vi "仪器版本写入.vi"(8 "error in (no error)":errorcluster caption="错误输入（无错误）", 10 "仪器版本":T1, 11 "SingleStepTestV3 输入":refnum<class "SingleStepTestV3.lvclass">) -> (0 "error out":errorcluster caption="错误输出", 3 "SingleStepTestV3 输出":refnum<class "SingleStepTestV3.lvclass">)   [LabVIEW 2022 SP3, in "SingleStepTestV3.lvlib" / "SingleStepTestV3.lvclass"]
uses:
  SingleStepTestV3.lvclass
  SingleStepTestV3.lvclass/SingleStepTestV3.ctl
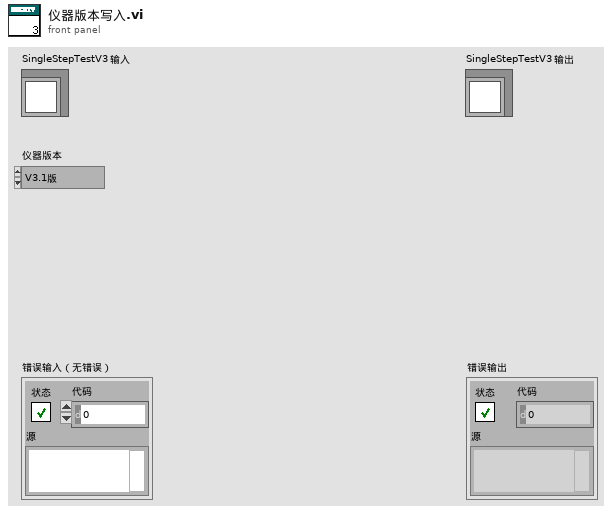
[diagram p1: front panel]
types:
  T1 = typedef "SingleStepTestV3.lvlib/SingleStepTestV3.lvclass/仪器版本.ctl" = enum16{"V3.1版", "V4版", "V3版", "V4.2版"}
  T2 = typedef "SingleStepTestV3.lvlib/SingleStepTestV3.lvclass/State Data.ctl" = cluster{"data":u16[], "仪器版本":T1}
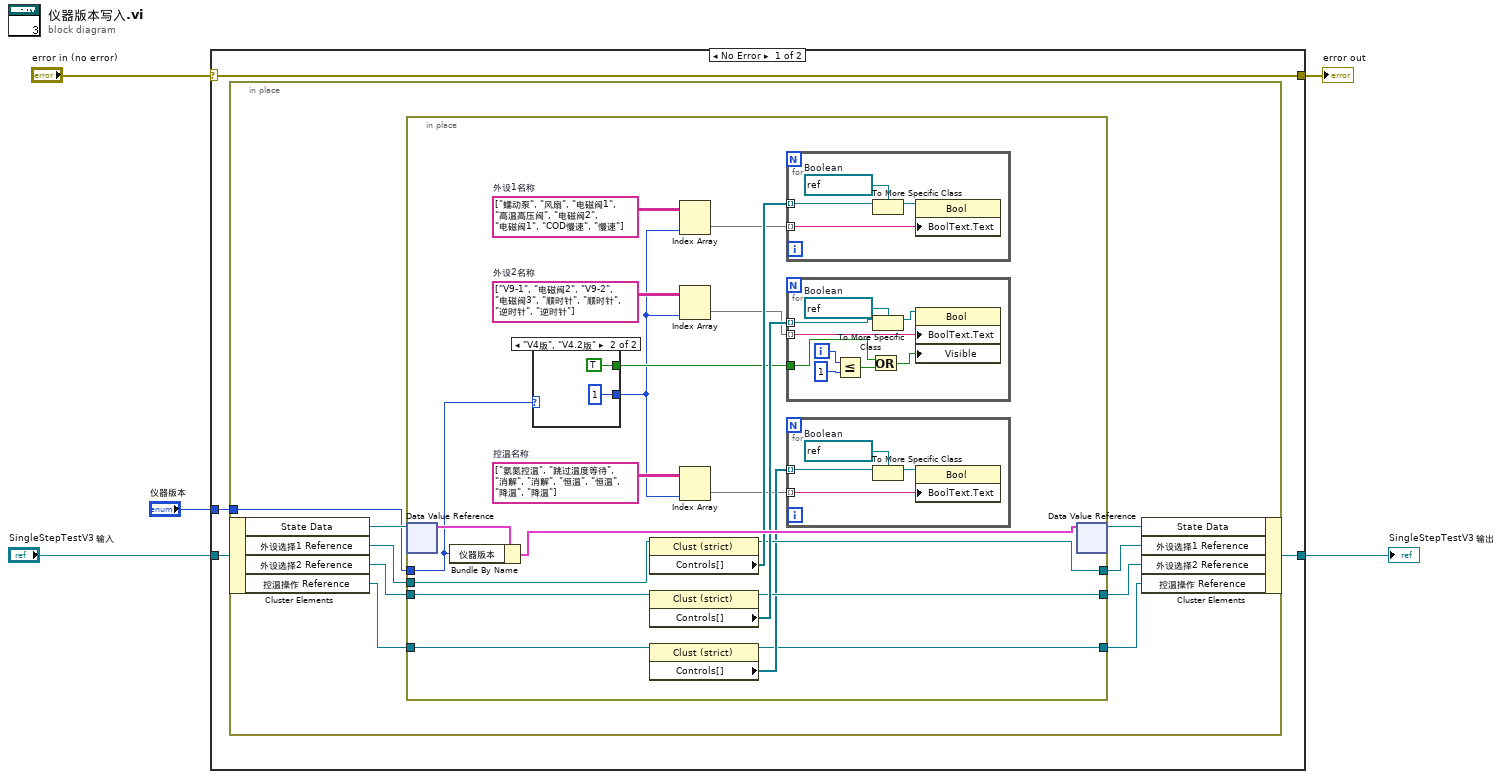
[diagram p0: block diagram]
diagram:
  n1 = case shown="No Error" "error in (no error)" {
    selector: "error in (no error)" -> [w9 w59]
    tunnel: [w9 w59] -> w4
    tunnel: [w7 w58] -> w2
    tunnel: "SingleStepTestV3 输入" -> [w8 w58]
    tunnel: "仪器版本" -> [w6 _]
    frame No Error {
      n2 = in-place {
        in-place-border: w6 -> [w16]
        n3 = in-place-cluster #1(w8) -> ("State Data"=w18:refnum<data-value>, "外设选择1 Reference"=w15:refnum<vi>, "外设选择2 Reference"=w14:refnum<vi>, "控温操作 Reference"=w11:refnum<vi>)
        n4 = in-place {
          in-place-border: w16 -> [w20]
          in-place-border: w15 -> [w36]
          in-place-border: w14 -> [w35]
          in-place-border: [w28] -> w13
          in-place-border: [w27] -> w12
          in-place-border: w11 -> [w26]
          in-place-border: [w22] -> w10
          w24 = string[][] [["氨氮控温", "跳过温度等待"], ["消解", "消解"], ["恒温", "恒温"], ["降温", "降温"]]  # 控温名称
          w30 = string[][] [["V9-1", "电磁阀2"], ["V9-2", "电磁阀3"], ["顺时针", "顺时针"], ["逆时针", "逆时针"]]  # 外设2名称
          w33 = string[][] [["蠕动泵", "风扇"], ["电磁阀1", "高温高压阀"], ["电磁阀2", "电磁阀1"], ["COD慢速", "慢速"]]  # 外设1名称
          n5 = in-place-dvr #2(w18) -> (w38:T2)  [unwired: 1 out]
          n6 = Bundle By Name(cluster=w38, "仪器版本"=w20) -> (w37:T2)
          n7 = case shown="\"V4版\", \"V4.2版\"" w20 {
            tunnel: [_ TRUE] -> w21
            tunnel: [_ 1] -> w19
            frame "V3.1版", Default {
            }
            frame "V4版", "V4.2版" {
            }
          }
          n8 = property class="Clust (strict)"(reference=w36) -> (reference out=w28:refnum<vi>, "Controls[]"=w34:refnum<vi>[])  [unwired: 1 in, 1 out]
          n9 = property class="Clust (strict)"(reference=w35) -> (reference out=w27:refnum<vi>, "Controls[]"=w31:refnum<vi>[])  [unwired: 1 in, 1 out]
          n10 = property class="Clust (strict)"(reference=w26) -> (reference out=w22:refnum<vi>, "Controls[]"=w25:refnum<vi>[])  [unwired: 1 in, 1 out]
          n11 = Index Array(array=w33, index (col)=w19) -> (element=w32:string[])  [unwired: 1 in]
          n12 = Index Array(array=w30, index (col)=w19) -> (element=w29:string[])  [unwired: 1 in]
          n13 = Index Array(array=w24, index (col)=w19) -> (element=w23:string[])  [unwired: 1 in]
          n14 = for {
            tunnel: w34 -> [w57] mode=indexing
            tunnel: w32 -> [w54] mode=indexing
            w55 = refnum<vi> refnum  # Boolean
            n15 = To More Specific Class(target class=w55, reference=w57) -> (specific class reference=w56:refnum<vi>)  [unwired: 1 in, 1 out]
            n16 = property class="Bool"(reference=w56, "BoolText.Text"=w54) -> ()  [unwired: 1 in, 2 out]
          }
          n17 = for {
            tunnel: w31 -> [w53] mode=indexing
            tunnel: w29 -> [w50] mode=indexing
            tunnel: w21 -> [w46]
            i -> [w49]
            w51 = refnum<vi> refnum  # Boolean
            n18 = Less Or Equal?(x=w49, y=1) -> (x <= y?=w47:bool)
            n19 = Or(x=w46, y=w47) -> (x .or. y?=w45:bool)
            n20 = To More Specific Class(target class=w51, reference=w53) -> (specific class reference=w52:refnum<vi>)  [unwired: 1 in, 1 out]
            n21 = property class="Bool"(reference=w52, "BoolText.Text"=w50, "Visible"=w45) -> ()  [unwired: 1 in, 2 out]
          }
          n22 = for {
            tunnel: w25 -> [w44] mode=indexing
            tunnel: w23 -> [w41] mode=indexing
            w42 = refnum<vi> refnum  # Boolean
            n23 = To More Specific Class(target class=w42, reference=w44) -> (specific class reference=w43:refnum<vi>)  [unwired: 1 in, 1 out]
            n24 = property class="Bool"(reference=w43, "BoolText.Text"=w41) -> ()  [unwired: 1 in, 2 out]
          }
          n25 = in-place-dvr #2(w37) -> (w17:refnum<data-value>)  [unwired: 1 out]
        }
        n26 = in-place-cluster #1("State Data"=w17, "外设选择1 Reference"=w13, "外设选择2 Reference"=w12, "控温操作 Reference"=w10) -> (w7:refnum<class "SingleStepTestV3.lvclass">)
      }
    }
    frame Error {
    }
  }
  "error out" <- w4
  "SingleStepTestV3 输出" <- w2
